vi "Add Tip Offset.vi"(11 "XYZTheta":dbl[](array[numeric])) -> (3 "XYZTheta":dbl[](array[numeric]))   [LabVIEW 2021, in "Dispense.lvclass"]
uses:
  Dispense.lvclass
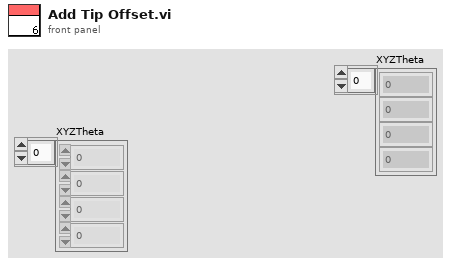
[diagram p1: front panel]
types:
  T1 = typedef "File Paths.ctl" = cluster{"Glue Pattern Folder":path, "Carrier Tray Folder":path, "Pick Up Tool Fixture Folder":path, "Components Folder":path, "Bellows Tool Offset.txt":path, "Pick Up Tool Offset.txt":path, "Dispense Tip Offset.txt":path, "Log Files":path, "Gantry Assembly Map.txt":path, "Syringe and offset map.txt":path, "Controllers Folder":path, "Local dbase config":path}
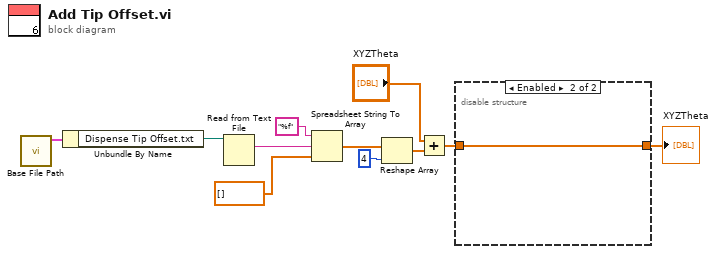
[diagram p0: block diagram]
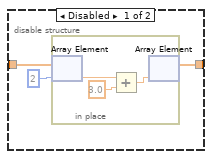
[diagram p2: hidden frame]
diagram:
  n1 = call "Base File Path.vi"() -> ("Paths Out"=w10:T1)  [unwired: 11 in]
  n2 = Unbundle By Name(w10) -> ("Dispense Tip Offset.txt"=w11:path)
  n3 = Read from Text File(file (use dialog)=w11) -> (text=w8:string)  [unwired: 3 in, 3 out]
  n4 = Spreadsheet String To Array(format string="%f", spreadsheet string=w8, array type (2D Dbl)=dbl[] []) -> (array=w4:dbl[])  [unwired: 1 in]
  n5 = Reshape Array(w4, 4 ("dimension size")) -> (w5:dbl[])
  n6 = Add(x="XYZTheta", y=w5) -> (x+y=w2:dbl[])
  n7 = disable-structure shown="Enabled" {
    disable-tunnel: w2 -> [w13 w18]
    disable-tunnel: [w12 w18] -> w1
    frame Disabled {
      n8 = in-place {
        n9 = in-place-array #1(w13, 2) -> (w17:dbl)
        n10 = Add(x=w17, y=3.0) -> (x+y=w16:dbl)
        n11 = in-place-array #1(w16) -> (w12:dbl[])  [unwired: 1 out]
      }
    }
    frame Enabled {
    }
  }
  "XYZTheta" <- w1
